vi "Confirm Disasters.vi"() -> (3 "Enable Disasters":bool)   [LabVIEW 2019]
panel:
  in  "Confirmation Text":string
  in  "Cancel":bool
  in  "Enable":bool
  out "Text":string="Disasters will mess up wiring, destroy code, and potentially corrupt VIs or the LabVIEW installation.\n\nEnsure your code is saved, committed, and backed up before proceeding! Type disasters in the box below to continue."
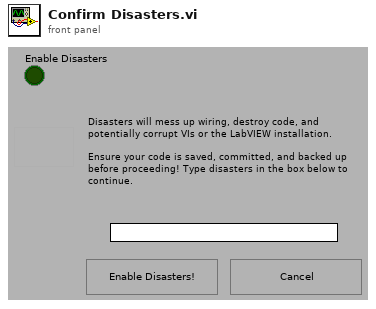
[diagram p1: front panel]
types:
  T1 = enum8{"Enabled", "Disabled", "Disabled and Grayed Out"}
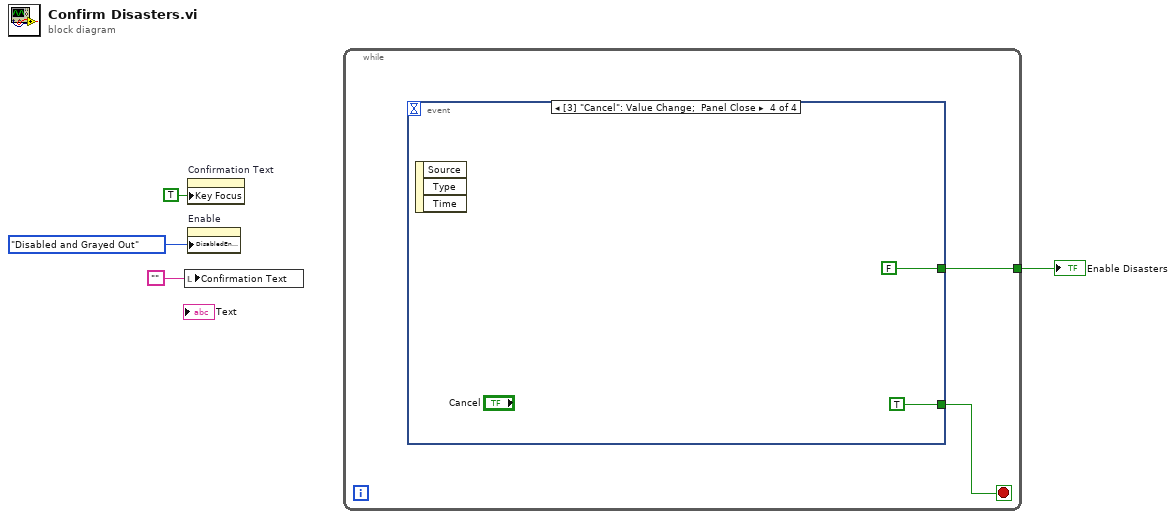
[diagram p0: block diagram]
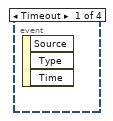
[diagram p2: hidden frame]
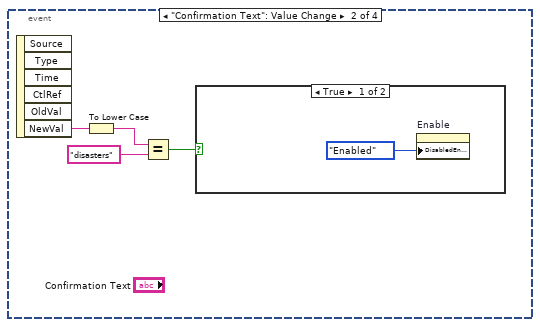
[diagram p3: hidden frame]
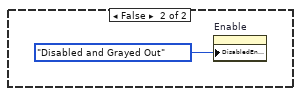
[diagram p4: hidden frame]
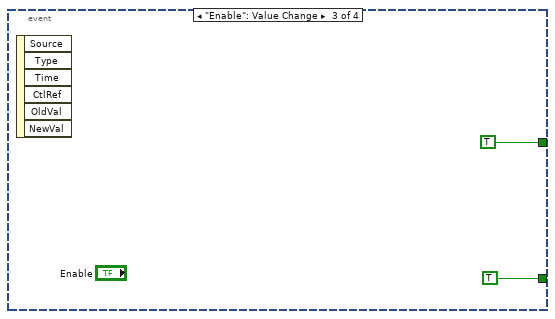
[diagram p5: hidden frame]
diagram:
  n1 = local write "Confirmation Text"("") -> ()
  n2 = property on="Confirmation Text" class="Str"("Key Focus"=TRUE) -> ()  [unwired: 2 in, 2 out]
  n3 = property on="Enable" class="Bool"("DisabledEnum"=T1."Disabled and Grayed Out" ("Disabled")) -> ()  [unwired: 2 in, 2 out]
  n4 = while {
    tunnel: [w6] -> w1
    stop <- w5 stop-if-true
    n5 = event shown="[3] \"Cancel\": Value Change;  Panel Close" {
      selector: _ -> [_ _ _ _]
      dyn-events: _ -> [_ _ _ _]
      timeout: _ -> [_ _ _ _]
      tunnel: [_ _ TRUE FALSE] -> w6
      tunnel: [_ _ TRUE TRUE] -> w5
      event Timeout {
        n6 = event-data() -> ()  [unwired: 1 in, 3 out]
      }
      event "Confirmation Text": Value Change {
        n7 = event-data() -> ("NewVal"=w10:string)  [unwired: 1 in, 5 out]
        n8 = To Lower Case(string=w10) -> (all lower case string=w9:string)
        n9 = Equal?(x=w9, y="disasters") -> (x = y?=w7:bool)
        n10 = case shown="True" w7 {
          frame True {
            n11 = property on="Enable" class="Bool"("DisabledEnum"=T1."Enabled" ("Disabled")) -> ()  [unwired: 2 in, 2 out]
          }
          frame False {
            n12 = property on="Enable" class="Bool"("DisabledEnum"=T1."Disabled and Grayed Out" ("Disabled")) -> ()  [unwired: 2 in, 2 out]
          }
        }
      }
      event "Enable": Value Change {
        n13 = event-data() -> ()  [unwired: 1 in, 6 out]
      }
      event "Cancel": Value Change; Panel Close {
        n14 = event-data() -> ()  [unwired: 1 in, 3 out]
      }
    }
  }
  "Enable Disasters" <- w1
